vi "Write Auto Iteration Notification.vi"(8 "error in (no error)":errorcluster, 10 "Auto Iteration Notification":bool, 11 "Iterator NR Actor in":refnum<class "Iterator NR Actor.lvclass">) -> (0 "error out":errorcluster, 3 "Iterator NR Actor out":refnum<class "Iterator NR Actor.lvclass">)   [LabVIEW 2023, in "Iterator Actor.lvlib" / "Iterator NR Actor.lvclass"]
uses:
  Iterator NR Actor.lvclass
  Iterator NR Actor.lvclass/Iterator NR Actor.ctl
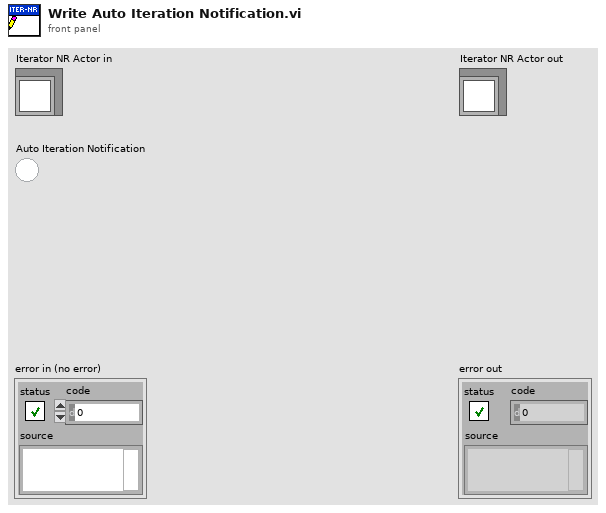
[diagram p1: front panel]
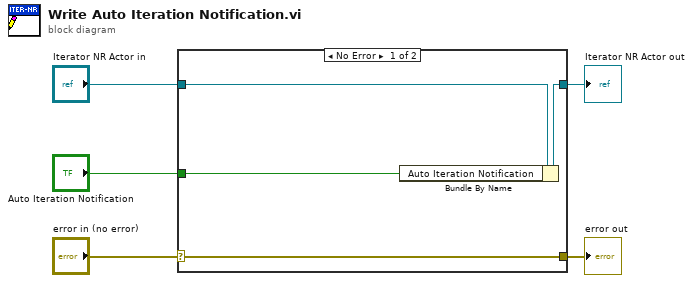
[diagram p0: block diagram]
diagram:
  n1 = case shown="No Error" "error in (no error)" {
    selector: "error in (no error)" -> [w9 w10]
    tunnel: [w9 w10] -> w4
    tunnel: [w7 w11] -> w2
    tunnel: "Iterator NR Actor in" -> [w8 w11]
    tunnel: "Auto Iteration Notification" -> [w6 _]
    frame No Error {
      n2 = Bundle By Name(cluster=w8, "Auto Iteration Notification"=w6) -> (w7:refnum<class "Iterator NR Actor.lvclass">)
    }
    frame Error {
    }
  }
  "error out" <- w4
  "Iterator NR Actor out" <- w2
